vi "VCS Set Ssi Abs Encoder Parameter.vi"(0 "axis in":cluster{"keyHandle":u32, "nodeId":u16}={"keyHandle"=0, "nodeId"=1}, 7 "SSI encoder":T1, 11 "error in (no error)":errorcluster) -> (4 "axis out":cluster{"keyHandle":u32, "nodeId":u16}={"keyHandle"=0, "nodeId"=1}, 15 "error out":errorcluster)   [LabVIEW 2018]
doc: "With function <B>VCS_SetSsiAbsEncoderParameter</B> it is possible to write all parameters for SSI absolute encoder."
uses:
  Resources/EposCmd64.dll
  Resources/EposCmd.dll
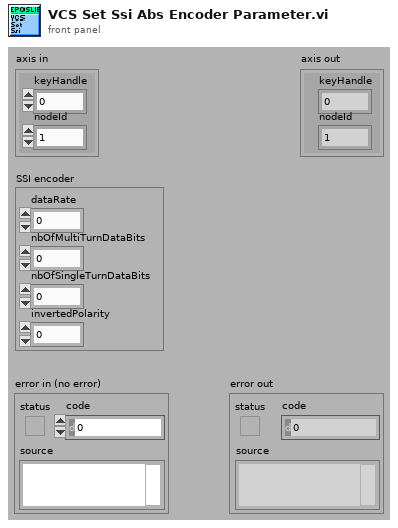
[diagram p1: front panel]
types:
  T1 = cluster{"dataRate":u16, "nbOfMultiTurnDataBits":u16, "nbOfSingleTurnDataBits":u16, "invertedPolarity":i32}
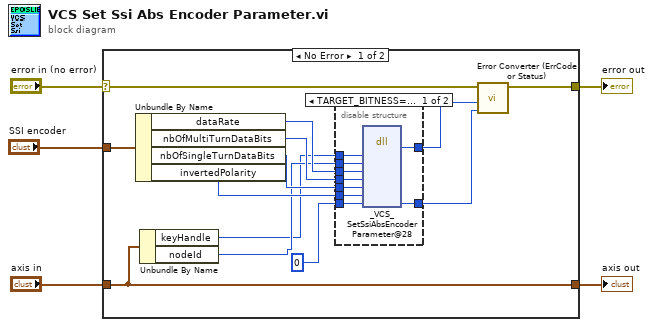
[diagram p0: block diagram]
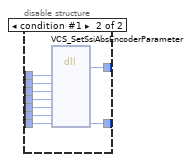
[diagram p2: hidden frame]
diagram:
  n1 = case shown="No Error" "error in (no error)" {
    selector: "error in (no error)" -> [w16 w37]
    tunnel: "axis in" -> [w18 w38]
    tunnel: [w18 w38] -> w4
    tunnel: [w17 w37] -> w3
    tunnel: "SSI encoder" -> [w15 _]
    frame No Error {
      n2 = Unbundle By Name(w15) -> ("dataRate"=w8:u16, "nbOfMultiTurnDataBits"=w9:u16, "nbOfSingleTurnDataBits"=w10:u16, "invertedPolarity"=w11:i32)
      n3 = Unbundle By Name(w18) -> ("keyHandle"=w6:u32, "nodeId"=w7:u16)
      n4 = disable-structure shown="TARGET_BITNESS==32, Standard" {
        disable-tunnel: [w27 w36] -> w14
        disable-tunnel: [w26 w35] -> w13
        disable-tunnel: u32 0 ("pErrorCode") -> [w25 w34]
        disable-tunnel: w11 -> [w24 w33]
        disable-tunnel: w10 -> [w23 w32]
        disable-tunnel: w9 -> [w22 w31]
        disable-tunnel: w8 -> [w21 w30]
        disable-tunnel: w7 -> [w20 w29]
        disable-tunnel: w6 -> [w19 w28]
        frame condition #0 (active) {
          n5 = dll-call lib="C:/Projeto em LabVIEW/EPOS-LabVIEW-Instrument-Driver-En/LabVIEW/maxon EPOS/Resources/EposCmd.dll" fn="_VCS_SetSsiAbsEncoderParameter@28"("KeyHandle"=w19, "NodeId"=w20, "DataRate"=w21, "NbOfMultiTurnDataBits"=w22, "NbOfSingleTurnDataBits"=w23, "InvertedPolarity"=w24, "pErrorCode"=w25) -> ("Rückgabetyp"=w27:i32, "pErrorCode"=w26:u32)  [unwired: 9 in, 2 out]
        }
        frame condition #1 {
          n6 = dll-call lib="C:/Sources/LabVIEW/maxon EPOS/Resources/EposCmd64.dll" fn="VCS_SetSsiAbsEncoderParameter" ("EposCmd.dll:_VCS_SetSsiAbsEncoderParameter@28")("KeyHandle"=w28, "NodeId"=w29, "DataRate"=w30, "NbOfMultiTurnDataBits"=w31, "NbOfSingleTurnDataBits"=w32, "InvertedPolarity"=w33, "pErrorCode"=w34) -> ("Rückgabetyp"=w36:i32, "pErrorCode"=w35:u32)  [unwired: 9 in, 2 out]
        }
      }
      n7 = call "Error Converter (ErrCode or Status).vi"("error code"=w13, "return type"=w14, "error in (no error)"=w16) -> ("error out"=w17:errorcluster)  [unwired: 7 in]
    }
    frame Error {
    }
  }
  "error out" <- w3
  "axis out" <- w4
